vi "LL VISA Write.vi"(7 "format string":string, 8 "error in (no error)":errorcluster, 10 "unsigned byte array":u8[](array[numeric]), 11 "LED Matrix in":refnum<class "LED Matrix.lvclass">) -> (0 "error out":errorcluster, 3 "LED Matrix out":refnum<class "LED Matrix.lvclass">)   [LabVIEW 2026, in "LED Matrix.lvlib" / "LED Matrix.lvclass"]
uses:
  LED Matrix.lvclass
  LED Matrix.lvclass/LED Matrix.ctl
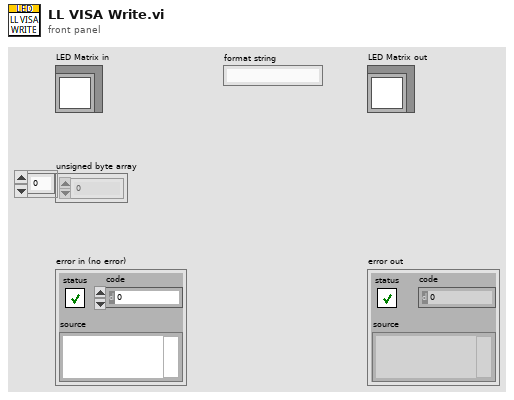
[diagram p1: front panel]
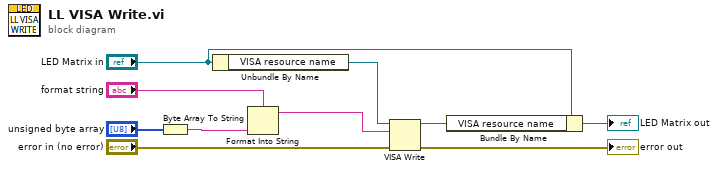
[diagram p0: block diagram]
diagram:
  n1 = Byte Array To String(unsigned byte array="unsigned byte array") -> (string=w10:string)
  n2 = Unbundle By Name("LED Matrix in") -> ("VISA resource name"=w7:refnum<visa-resource-name>)
  n3 = Format Into String(format string="format string", w10) -> (resulting string=w9:string)  [unwired: 2 in, 1 out]
  n4 = VISA Write(VISA resource name=w7, write buffer=w9, error in (no error)="error in (no error)") -> (VISA resource name out=w5:refnum<visa-resource-name>, error out=→"error out":errorcluster)  [unwired: 1 out]
  n5 = Bundle By Name(cluster="LED Matrix in", "VISA resource name"=w5) -> (→"LED Matrix out":refnum<class "LED Matrix.lvclass">)
